vi "Launcher.vi"   [LabVIEW 2020]
uses:
  Controller/Controller.lvclass
  C:/Program Files (x86)/National Instruments/LabVIEW 2020/vi.lib/ActorFramework/Actor/Actor.lvclass
  <vilib>/ActorFramework/Actor/Actor.lvclass
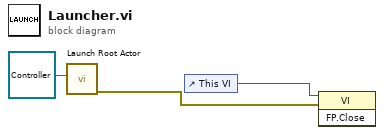
[diagram p0: block diagram]
diagram:
  n1 = call <vilib>:"Launch Root Actor.vi"("Actor"=refnum<class "Controller.lvclass"> refnum ("Controller.lvlib:Controller.lvclass")) -> ("error out"=w1:errorcluster)  [unwired: 9 in, 1 out]
  n2 = control-ref of="This VI"() -> (w2:refnum<vi>)
  n3 = invoke class="VI" method="FP.Close"(reference=w2, error in=w1) -> ()  [unwired: 1 in, 3 out]
